vi "removeLeadingZeros.vi"(11 "input":dbl[](array[numeric])) -> (3 "output":dbl[](array[numeric]))   [LabVIEW 2017]
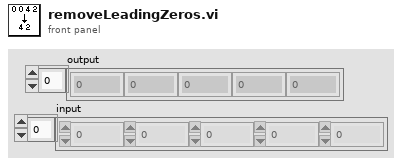
[diagram p1: front panel]
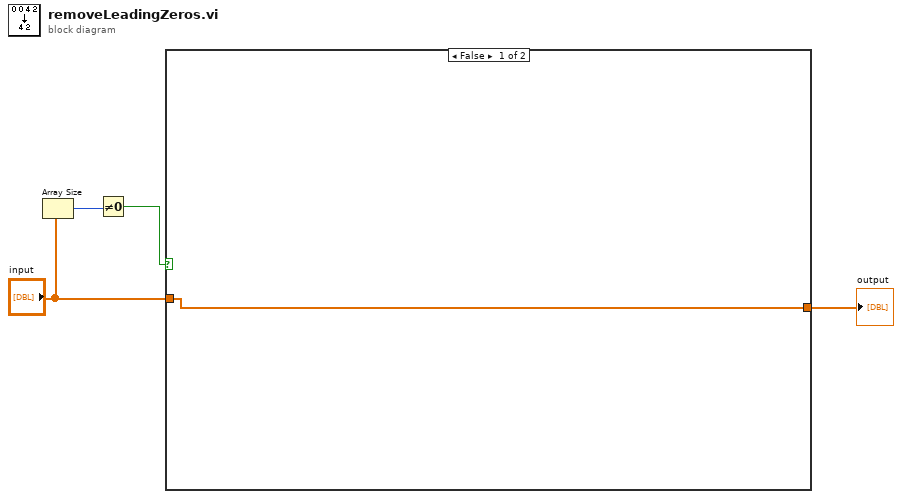
[diagram p0: block diagram]
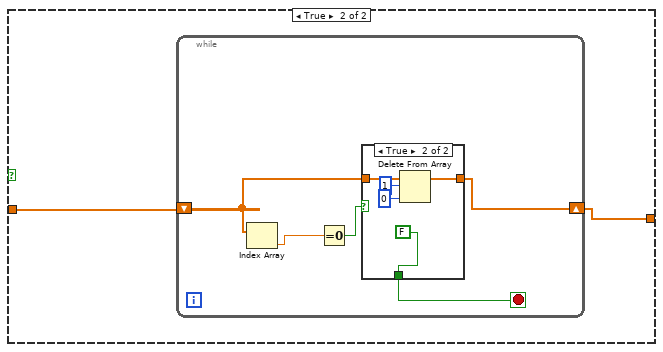
[diagram p2: hidden frame]
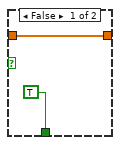
[diagram p3: hidden frame]
diagram:
  n1 = Array Size(array="input") -> (size(s)=w2:i32)
  n2 = Not Equal To 0?(x=w2) -> (x != 0?=w1:bool)
  n3 = case shown="False" w1 {
    tunnel: "input" -> [w5 w7]
    tunnel: [w5 w6] -> w4
    frame False {
    }
    frame True {
      n4 = while {
        shift-right: [w9] -> w6
        shift-left: w7 -> [w10]
        stop <- w8 stop-if-true
        n5 = Index Array(array=w10) -> (element=w12:dbl)  [unwired: 1 in]
        n6 = Equal To 0?(x=w12) -> (x = 0?=w11:bool)
        n7 = case shown="True" w11 {
          tunnel: [w14 w19] -> w9
          tunnel: w10 -> [w14 w18]
          tunnel: [TRUE FALSE] -> w8
          frame False {
          }
          frame True {
            n8 = Delete From Array(array=w18, length=1, index=0) -> (array with subset deleted=w19:dbl[])  [unwired: 1 out]
          }
        }
      }
    }
  }
  "output" <- w4
